vi "Drive Controller.vi"(8 "error in":errorcluster) -> ()   [LabVIEW 2020]
doc: "This VI executes continuously carrying out the current operation and responding to updates or new operation requests. It will often contain the timing or control code that is difficult to place directly in TeleOp. This VI generally opens all sensors and motors and isolates the rest of the robot code from knowing implementation details of how the operations are carried out."
uses:
  <vilib>/Rock Robotics/WPI/Framework/Completion Status.ctl
  Drive Setpoints.ctl
  Drive Operations.ctl
  <vilib>/Rock Robotics/WPI/ThirdParty/Phoenix-LabVIEW/Motor Controller/Controls/CTRE_Phoenix_MotorControl_ControlMode.ctl
  <vilib>/Rock Robotics/WPI/ThirdParty/REV Robotics/REVLib/Typedef/Spark MAX Control Type.ctl
panel:
  in  "Interactive Values":T1
  in  "Buttons":cluster{"Execute Cmd":bool, "Abort Cmd":bool}
  out "Command Timing":cluster{"Start Time (ms)":u32, "Iterations":i32}
  out "Status":T3
  out "Current\nCmd":string
  # "Tip: The graph shows the motor setpoints. It may also be helpful to observe inputs and sensor values.\nYou may also want to display tuning or debugging controls."
  # "Interactive Command: You may fill in the settings for a command\nand schedule it with the Execute button. You can observe and abort\nany command while fine tuning the code for the controller."
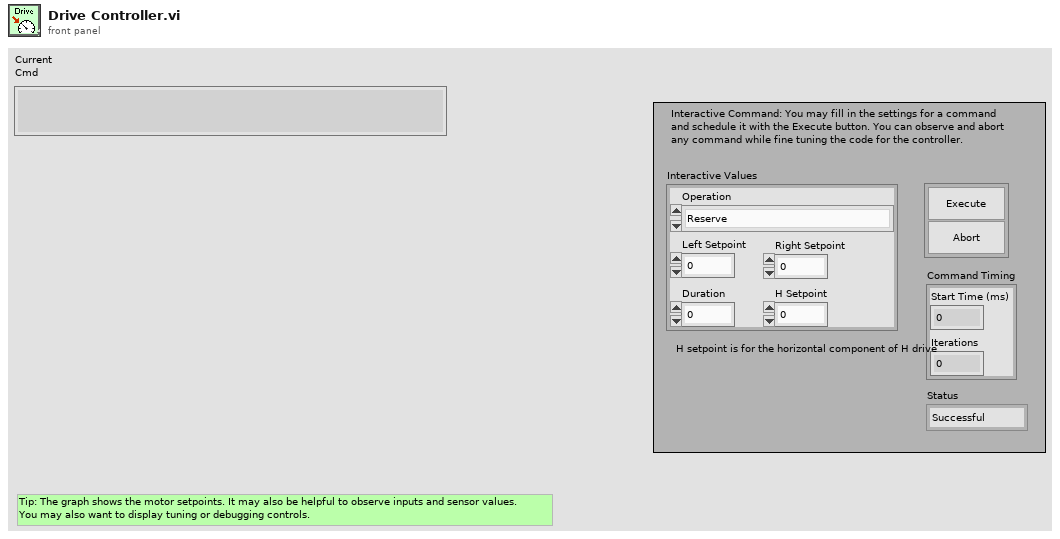
[diagram p1: front panel]
types:
  T1 = typedef "Drive Setpoints.ctl" = cluster{"Operation":T2, "Left Setpoint":dbl, "Right Setpoint":dbl, "Duration":dbl, "H Setpoint":dbl}
  T2 = typedef "Drive Operations.ctl" = enum16{"Reserve", "Read Current", "Immediate", "H-Drive Immediate", "Drive for Time", "Drive for Distance"}
  T3 = typedef "Completion Status.ctl" = enum16{"Successful", "Aborted", "Incomplete"}
  T4 = enum16{"FollowerType_PercentOutput", "FollowerType_AuxOutput1"}
  T5 = typedef "WPI_MotorControlDeviceRef.ctl" = cluster{"DeviceStatus":errorcluster, "Type":T6, "PWM":cluster{"PWM Channel":T7, "DeadBand":T8}, "CAN":cluster{"Device Number":u8, "SetOutput VI Ref":variant, "GetOutput VI Ref":variant, "Enable VI Ref":variant, "Disable VI Ref":variant, "Data":variant}, "Invert":bool, "DIO PWM":cluster{"PWM \"Enable\" Channel":T7, "DIOChannel":T9, "PWM Rate":dbl}}
  T6 = typedef "WPI_MotorControlType.ctl" = enum16{"PWM", "CAN", "DIO PWM"}
  T7 = typedef "FPGA_DIOPWMChannel.ctl" = enum8{"PWM 0", "PWM 1", "PWM 2", "PWM 3", "PWM 4", "PWM 5", "PWM 6", "PWM 7", "PWM 8", "PWM 9", "PWM MXP 0", "PWM MXP 1", "PWM MXP 2", "PWM MXP 3", "PWM MXP 4", "PWM MXP 5", "PWM MXP 6", "PWM MXP 7", "PWM MXP 8", "PWM MXP 9", "Invalid"}
  T8 = typedef "WPI_PWMDeadband.ctl" = cluster{"Name":string, "maxPositivePwm":i32, "minPositivePwm":i32, "centerPwm":i32, "maxNegativePwm":i32, "minNegativePwm":i32, "angularRange":u16}
  T9 = typedef "FPGA_DIOChannel.ctl" = enum8{"DIO 0", "DIO 1", "DIO 2", "DIO 3", "DIO 4", "DIO 5", "DIO 6", "DIO 7", "DIO 8", "DIO 9", "DIO MXP 0", "DIO MXP 1", "DIO MXP 2", "DIO MXP 3", "DIO MXP 4", "DIO MXP 5", "DIO MXP 6", "DIO MXP 7", "DIO MXP 8", "DIO MXP 9", "DIO MXP 10", "DIO MXP 11", "DIO MXP 12", "DIO MXP 13", "DIO MXP 14", "DIO MXP 15", "SPI Port CS1", "SPI Port CS2", "SPI Port CS3", "SPI Port MISO", "SPI Port MOSI", "Invalid"}
  T10 = typedef "Command Status Info.ctl" = cluster{"Name":string, "Status":T3, "notifier out":T11}
  T11 = typedef "Completion Notifier.ctl" = refnum<notifier>
  T12 = cluster{"SubSystem Data":T1, cluster{"Start Time (ms)":u32, "Iterations":i32}, cluster{"Command Info":T10, "Description":string, "Default Command":T1, "queue out":refnum<queue>, "Subsystem Name":string}}
  T13 = typedef "Spark MAX Control Type.ctl" = enum16{"Percent VBus", "Voltage", "Velocity", "Position", "Smart Motion", "Current", "Smart Velocity"}
  T14 = typedef "CTRE_Phoenix_MotorControl_ControlMode.ctl" = u16
  T15 = cluster{"SubSystem Data":T1, cluster{"Start Time (ms)":u32, "Iterations":i32}, "Default Command Arguments":cluster{"Command Info":T10, "Description":string, "Default Command":T1, "queue out":refnum<queue>, "Subsystem Name":string}}
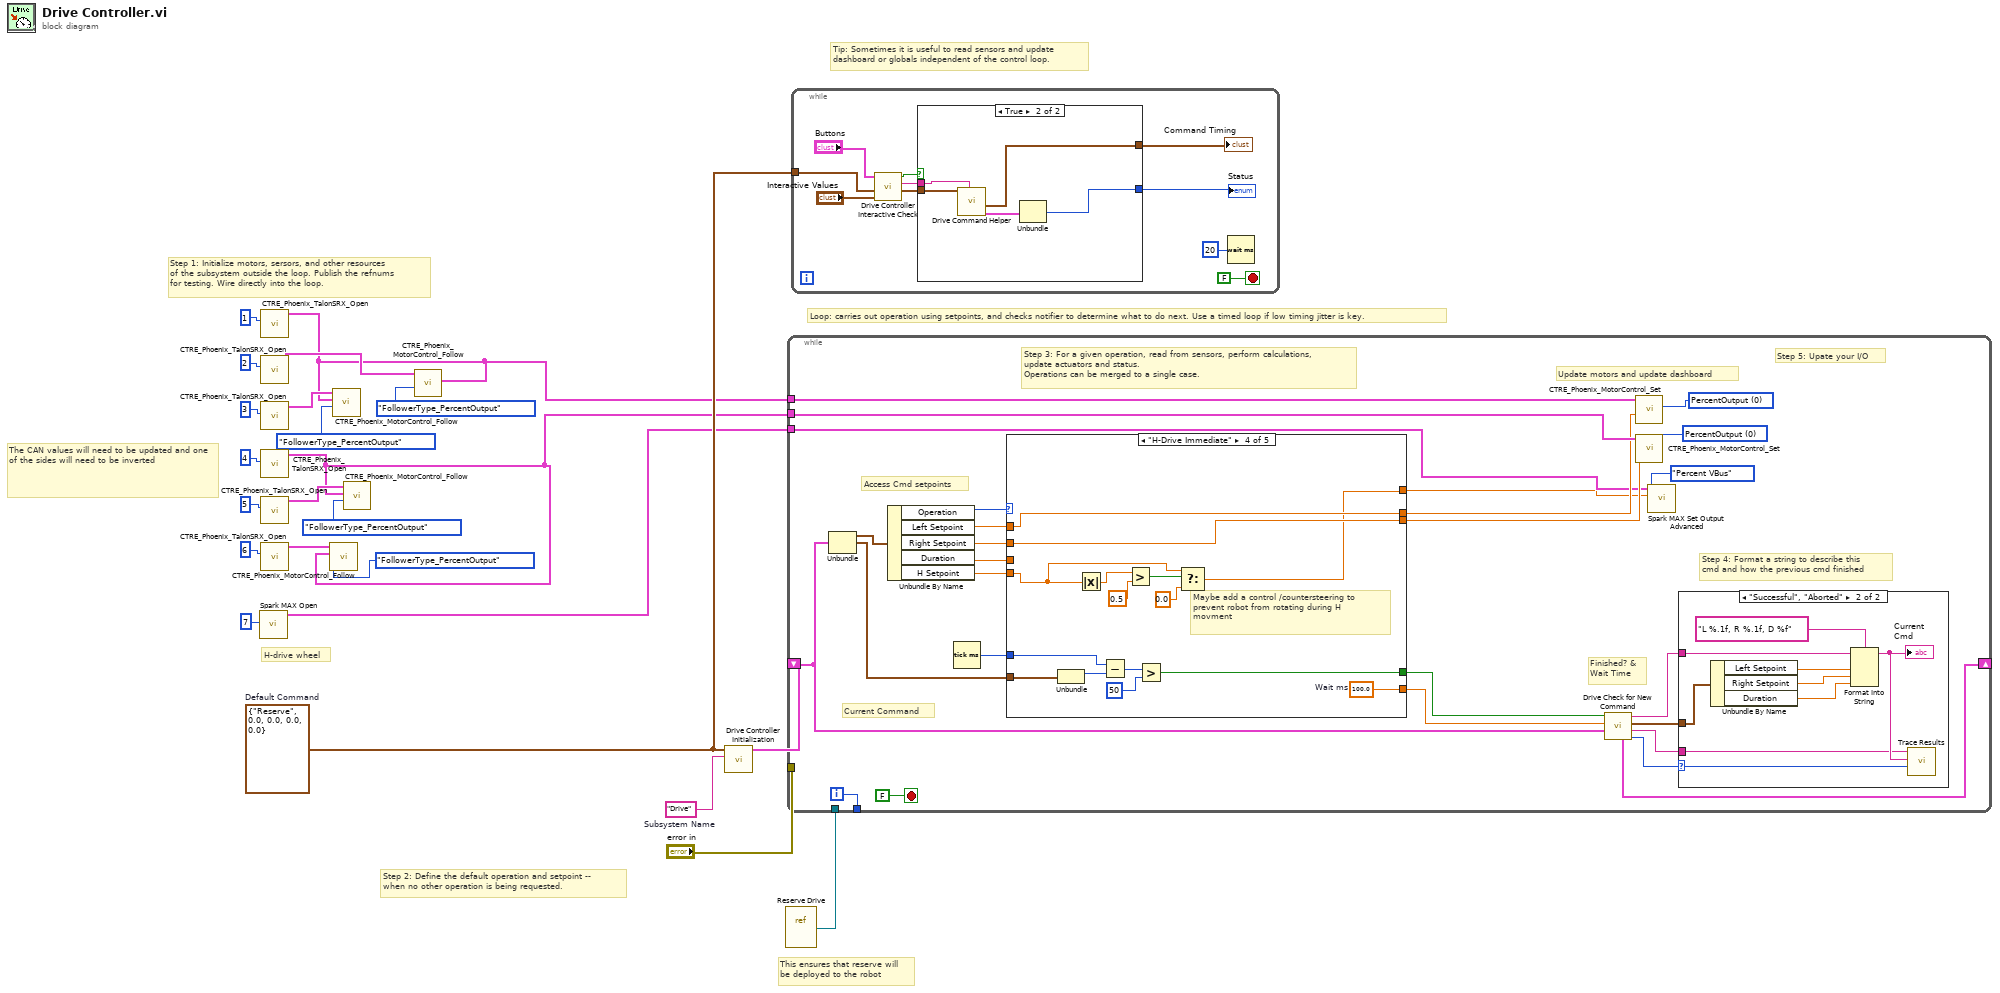
[diagram p0: block diagram]
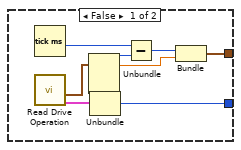
[diagram p2: hidden frame]
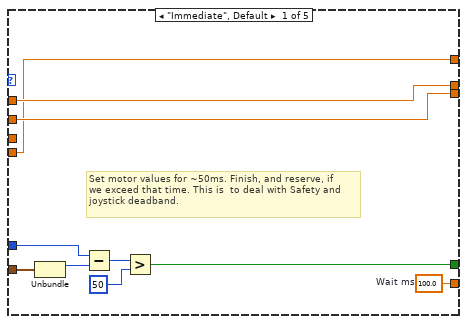
[diagram p4: hidden frame]
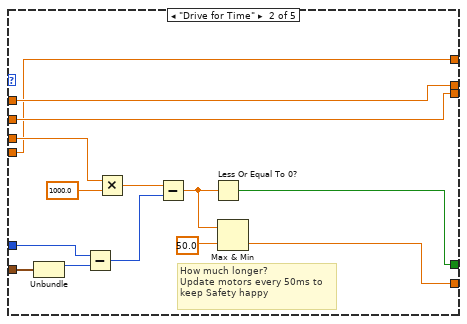
[diagram p5: hidden frame]
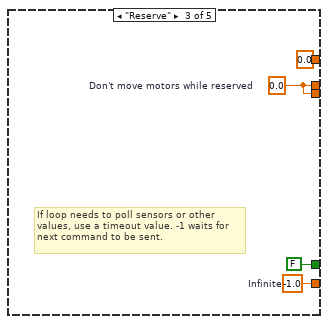
[diagram p6: hidden frame]
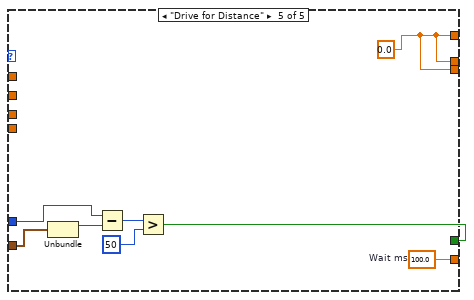
[diagram p7: hidden frame]
diagram:
  w19 = T1 {"Operation"=enum."Reserve", "Left Setpoint"=0.0, "Right Setpoint"=0.0, "Duration"=0.0, "H Setpoint"=0.0}  # Default Command
  w23 = "Drive"  # Subsystem Name
  # "H-drive wheel"
  # "The CAN values will need to be updated and one of the sides will need to be inverted"
  # "This ensures that reserve will\nbe deployed to the robot"
  # "Tip: Sometimes it is useful to read sensors and update\ndashboard or globals independent of the control loop."
  # "Step 2: Define the default operation and setpoint --\nwhen no other operation is being requested."
  # "Step 1: Initialize motors, sersors, and other resources\nof the subsystem outside the loop. Publish the refnums\nfor testing. Wire directly into the loop."
  # "Loop: carries out operation using setpoints, and checks notifier to determine what to do next. Use a timed loop if low timing jitter is key."
  n1 = call <vilib>:"Spark MAX Open.vi"("Device Number"=u8 7) -> ("MotorControlDeviceRef"=w2:T5)  [unwired: 9 in, 1 out]
  n2 = call <vilib>:"CTRE_Phoenix_TalonSRX_Open.vi"("Device Number"=u8 1) -> ("PhoenixMotorControlDevRef"=w9:T5)  [unwired: 9 in, 1 out]
  n3 = call <vilib>:"CTRE_Phoenix_TalonSRX_Open.vi"("Device Number"=u8 2) -> ("PhoenixMotorControlDevRef"=w12:T5)  [unwired: 9 in, 1 out]
  n4 = call <vilib>:"CTRE_Phoenix_TalonSRX_Open.vi"("Device Number"=u8 3) -> ("PhoenixMotorControlDevRef"=w10:T5)  [unwired: 9 in, 1 out]
  n5 = call <vilib>:"CTRE_Phoenix_TalonSRX_Open.vi"("Device Number"=u8 4) -> ("PhoenixMotorControlDevRef"=w1:T5)  [unwired: 9 in, 1 out]
  n6 = call <vilib>:"CTRE_Phoenix_TalonSRX_Open.vi"("Device Number"=u8 5) -> ("PhoenixMotorControlDevRef"=w7:T5)  [unwired: 9 in, 1 out]
  n7 = call <vilib>:"CTRE_Phoenix_TalonSRX_Open.vi"("Device Number"=u8 6) -> ("PhoenixMotorControlDevRef"=w5:T5)  [unwired: 9 in, 1 out]
  n8 = call <vilib>:"CTRE_Phoenix_MotorControl_Follow.vi"("FollowerType"=T4."FollowerType_PercentOutput", "Master Controller to Follow"=w1, "PhoenixMotorControlDevRef"=w5) -> ()  [unwired: 7 in, 2 out]
  n9 = call <vilib>:"CTRE_Phoenix_MotorControl_Follow.vi"("FollowerType"=T4."FollowerType_PercentOutput", "Master Controller to Follow"=w9, "PhoenixMotorControlDevRef"=w10) -> ()  [unwired: 7 in, 2 out]
  n10 = call <vilib>:"CTRE_Phoenix_MotorControl_Follow.vi"("FollowerType"=T4."FollowerType_PercentOutput", "Master Controller to Follow"=w1, "PhoenixMotorControlDevRef"=w7) -> ()  [unwired: 7 in, 2 out]
  n11 = call <vilib>:"CTRE_Phoenix_MotorControl_Follow.vi"("FollowerType"=T4."FollowerType_PercentOutput", "Master Controller to Follow"=w9, "PhoenixMotorControlDevRef"=w12) -> ()  [unwired: 7 in, 2 out]
  n12 = call "Drive Controller Initialization.vi"("Subsystem Name"=w23, "Default Command"=w19) -> ("Current Command"=w21:T12)  [unwired: 9 in]
  n13 = vi-ref "Reserve Drive.vi"() -> (w20:refnum<vi>)
  n14 = while {
    shift-right: [w41] -> _
    shift-left: w21 -> [w34]
    tunnel: [w49] -> _
    tunnel: "error in" -> [_]
    tunnel: w20 -> [_]
    tunnel: w9 -> [w33]
    tunnel: w1 -> [w32]
    tunnel: w2 -> [w29]
    i -> [w49]
    stop <- FALSE stop-if-true
    w25 = T14 0 items=["PercentOutput"=0, "Position"=1, "Velocity"=2, "Current"=3, "Follower"=5, "MotionProfile"=6, "MotionMagic"=7, "MotionProfileArc"=10, "Disabled"=15] ("Control Mode")
    w26 = T14 0 items=["PercentOutput"=0, "Position"=1, "Velocity"=2, "Current"=3, "Follower"=5, "MotionProfile"=6, "MotionMagic"=7, "MotionProfileArc"=10, "Disabled"=15] ("Control Mode")
    # "Step 5: Upate your I/O"
    # "Step 4: Format a string to describe this\ncmd and how the previous cmd finished"
    # "Current Command"
    # "Update motors and update dashboard"
    # "Access Cmd setpoints"
    # "Finished? &\nWait Time"
    # "Step 3: For a given operation, read from sensors, perform calculations,\nupdate actuators and status.\nOperations can be merged to a single case."
    n15 = Unbundle(w34) -> ("SubSystem Data"=w48:T1, w35:cluster{"Start Time (ms)":u32, "Iterations":i32})  [unwired: 1 out]
    n16 = Unbundle By Name(w48) -> ("Operation"=w47:T2, "Left Setpoint"=w46:dbl, "Right Setpoint"=w45:dbl, "Duration"=w44:dbl, "H Setpoint"=w27:dbl)
    n17 = Tick Count (ms)() -> (millisecond timer value=w43:u32)
    n18 = case shown="\"H-Drive Immediate\"" w47 {
      tunnel: [w69 w71 w87 w88 w103] -> w40
      tunnel: [w62 w78 FALSE ("ignore previous (F)") w89 w104] -> w39
      tunnel: w35 -> [w61 w80 _ w90 w105]
      tunnel: [w68 w77 w85 w102 w110] -> w31
      tunnel: [w67 w76 w85 w101 w110] -> w30
      tunnel: w46 -> [w68 w77 _ w102 _]
      tunnel: w45 -> [w67 w76 _ w101 _]
      tunnel: w44 -> [_ w75 _ _ _]
      tunnel: w43 -> [w63 w74 _ w91 w106]
      tunnel: [w60 w70 0.0 ("Duration") w97 w110] -> w28
      tunnel: w27 -> [w60 w70 _ w96 _]
      frame "Immediate", Default {
        w69 = 100.0  # Wait ms
        # "Set motor values for ~50ms. Finish, and reserve, if\nwe exceed that time. This is  to deal with Safety and\njoystick deadband."
        n19 = Unbundle(w61) -> ("Start Time (ms)"=w64:u32)  [unwired: 1 out]
        n20 = Subtract(x=w63, y=w64) -> (x-y=w65:u32)
        n21 = Greater?(x=w65, y=u8 50 ("Left Motor")) -> (0:w62:bool)
      }
      frame "Drive for Time" {
        # "How much longer?\nUpdate motors every 50ms to\nkeep Safety happy"
        n22 = Unbundle(w80) -> ("Start Time (ms)"=w79:u32)  [unwired: 1 out]
        n23 = Subtract(x=w74, y=w79) -> (x-y=w83:u32)
        n24 = Multiply(x=w75, y=1000.0) -> (x*y=w82:dbl)
        n25 = Subtract(x=w82, y=w83) -> (x-y=w73:dbl)
        n26 = Less Or Equal To 0?(x=w73) -> (x <= 0?=w78:bool)
        n27 = Max & Min(x=w73, y=50.0) -> (min(x,y)=w71:dbl)  [unwired: 1 out]
      }
      frame "Reserve" {
        w85 = 0.0  # Don't move motors while reserved
        w87 = -1.0  # Infinite
        # "If loop needs to poll sensors or other\nvalues, use a timeout value. -1 waits for\nnext command to be sent."
      }
      frame "H-Drive Immediate" {
        w88 = 100.0  # Wait ms
        # "Maybe add a control /countersteering to prevent robot from rotating during H movment"
        n28 = Unbundle(w90) -> ("Start Time (ms)"=w92:u32)  [unwired: 1 out]
        n29 = Absolute Value(x=w96) -> (abs(x)=w100:dbl)
        n30 = Subtract(x=w91, y=w92) -> (x-y=w93:u32)
        n31 = Greater?(x=w100, y=0.5) -> (0:w98:bool)
        n32 = Greater?(x=w93, y=u8 50 ("Left Motor")) -> (0:w89:bool)
        n33 = Select(t=w96, s=w98, f=0.0) -> (s? t:f=w97:dbl)
      }
      frame "Drive for Distance" {
        w103 = 100.0  # Wait ms
        w110 = 0.0
        n34 = Unbundle(w105) -> ("Start Time (ms)"=w107:u32)  [unwired: 1 out]
        n35 = Subtract(x=w106, y=w107) -> (x-y=w108:u32)
        n36 = Greater?(x=w108, y=u8 50 ("Left Motor")) -> (0:w104:bool)
      }
    }
    n37 = call "Drive Check for New Command.vi"("input cluster"=w34, "Wait time (ms)"=w40, "Finished?"=w39) -> ("Completion"=w42:T3, "Subsystem Name"=w36:string, "Current Command"=w37:T1, "Initial Trace String"=w38:string, "Next Command"=w41:T15)  [unwired: 4 in]
    n38 = call <vilib>:"CTRE_Phoenix_MotorControl_Set.vi"("Output"=w31, "Control Mode"=w26, "PhoenixMotorControlDevRef"=w33) -> ()  [unwired: 7 in, 2 out]
    n39 = call <vilib>:"CTRE_Phoenix_MotorControl_Set.vi"("Output"=w30, "Control Mode"=w25, "PhoenixMotorControlDevRef"=w32) -> ()  [unwired: 7 in, 2 out]
    n40 = call <vilib>:"Spark MAX Set Output Advanced.vi"("Control Mode"=Spark_MAX_Control_Type."Percent VBus", "Setpoint"=w28, "MotorControlDevRef"=w29) -> ()  [unwired: 7 in, 2 out]
    n41 = case shown="\"Successful\", \"Aborted\"" w42 {
      selector: w42 -> [_ w59]
      tunnel: w38 -> [_ w54]
      tunnel: w37 -> [_ w55]
      tunnel: w36 -> [_ w51]
      frame "Incomplete", Default {
        # "Continuing current command"
      }
      frame "Successful", "Aborted" {
        # "Report and setup for next command"
        n42 = Unbundle By Name(w55) -> ("Left Setpoint"=w57:dbl, "Right Setpoint"=w58:dbl, "Duration"=w52:dbl)
        n43 = Format Into String(format string="L %.1f, R %.1f, D %f", initial string=w54, w57, w58, w52) -> (resulting string=w53:string)  [unwired: 1 in, 1 out]
        "Current\nCmd" <- w53
        n44 = call <vilib>:"Trace Results.vi"("Status of previous command"=w59, "Description"=w53, "Subsystem"=w51) -> ()  [unwired: 9 in]
      }
    }
  }
  n45 = while {
    tunnel: w19 -> [w112]
    stop <- FALSE stop-if-true
    n46 = call "Drive Controller Interactive Check.vi"("Interactive Command In"="Interactive Values", "Default Command"=w112, "Buttons"="Buttons") -> ("Interactive Command Out"=w114:T1, "Trace String"=w115:string, "Schedule"=w116:bool)  [unwired: 6 in]
    n47 = case shown="True" w116 {
      tunnel: [w125 w133] -> w117
      tunnel: [w124 w129] -> w118
      tunnel: w115 -> [_ w131]
      tunnel: w114 -> [_ w130]
      frame False {
        n48 = Tick Count (ms)() -> (millisecond timer value=w128:u32)
        n49 = call "Read Drive Operation.vi"() -> ("Command Info"=w122:T10, "SubSystem Data"=w121:T1)  [unwired: 9 in, 1 out]
        n50 = Unbundle(w121) -> ("Operation"=w126:T2, "Left Setpoint"=w123:dbl)  [unwired: 3 out]
        n51 = Unbundle(w122) -> ("Status"=w125:T3)  [unwired: 2 out]
        n52 = Subtract(x=w128, y=w126) -> (x-y=w127:u32)
        n53 = Bundle(w127, "Left Setpoint"=w123) -> (w124:cluster{u32, "Left Setpoint":dbl})  [unwired: 1 in]
      }
      frame True {
        n54 = call "Drive Command Helper.vi"("Description"=w131, "SubSystem Data"=w130) -> ("Command Info Out"=w132:T10, "Command Timing"=w129:cluster{"Start Time (ms)":u32, "Iterations":i32})  [unwired: 7 in, 1 out]
        n55 = Unbundle(w132) -> ("Status"=w133:T3)  [unwired: 2 out]
      }
    }
    "Status" <- w117
    "Command Timing" <- w118
    n56 = Wait (ms)(milliseconds to wait=u32 20) -> ()  [unwired: 1 out]
  }
